vi "Read Result Elements.vi"(8 "error in (no error)":errorcluster, 11 "csv-formatter in":refnum<class "csv-formatter.lvclass">) -> (0 "error out":errorcluster, 2 "Result Elements":T1=["Step Name", "Step Class", "Low Limit", "Measurement", "High Limit", "Comparison", "Duration"], 3 "csv-formatter out":refnum<class "csv-formatter.lvclass">)   [LabVIEW 2015, in "csv-formatter.lvclass"]
uses:
  csv-formatter.lvclass
  Config/Result Config.ctl
  csv-formatter.lvclass/csv-formatter.ctl
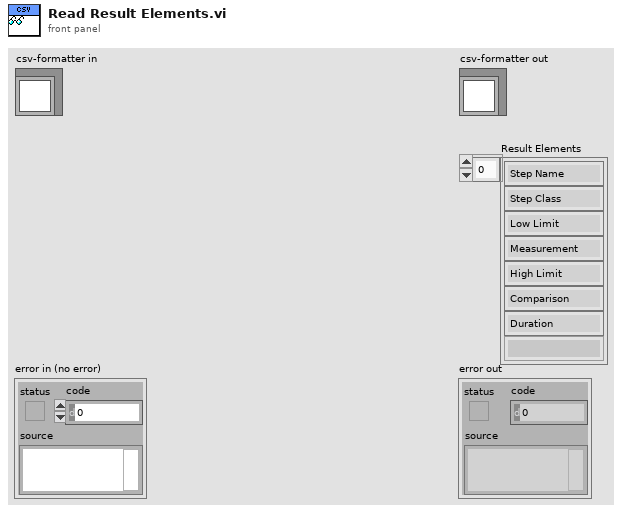
[diagram p1: front panel]
types:
  T1 = typedef "Result Config.ctl" = string[]
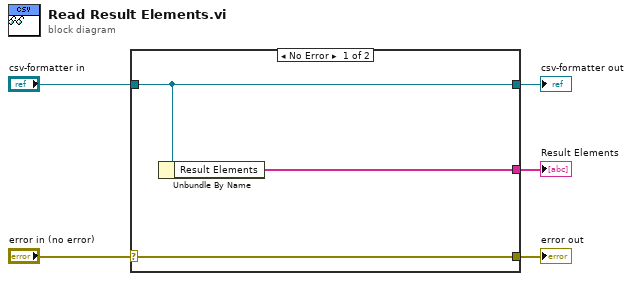
[diagram p0: block diagram]
diagram:
  n1 = case shown="No Error" "error in (no error)" {
    selector: "error in (no error)" -> [w8 w9]
    tunnel: [w8 w9] -> w4
    tunnel: [w7 w10] -> w2
    tunnel: "csv-formatter in" -> [w7 w10]
    tunnel: [w6 _] -> w1
    frame No Error {
      n2 = Unbundle By Name(w7) -> ("Result Elements"=w6:T1)
    }
    frame Error {
    }
  }
  "error out" <- w4
  "csv-formatter out" <- w2
  "Result Elements" <- w1
